vi "DAC PowerDown Step.vi"(5 "start label":string, 6 "DAC channel":u32, 7 "waveform name":string, 8 "error in":errorcluster, 11 "Digital sesssion":refnum<k15>) -> (0 "error out":errorcluster, 3 "Digital session out":refnum<k15>)   [LabVIEW 2021]
uses:
  <instrlib>/niDigital/niDigital.llb/niDigital Write Source Waveform (Broadcast U32).vi
  <instrlib>/niDigital/niDigital.llb/niDigital Burst Pattern (Pass Fail).vi
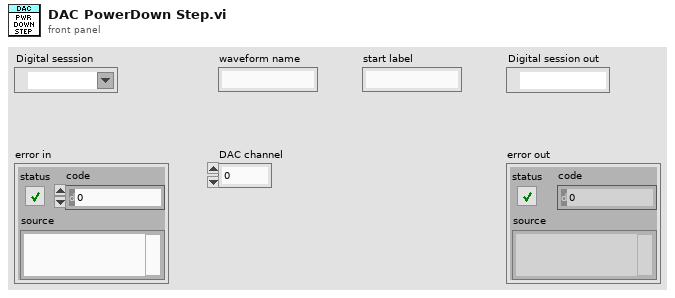
[diagram p1: front panel]
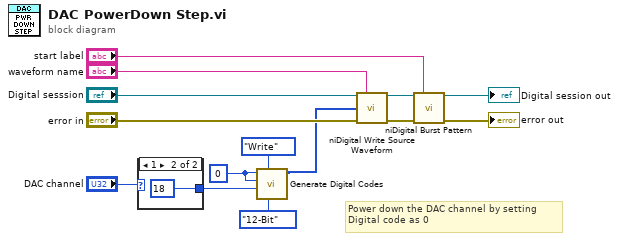
[diagram p0: block diagram]
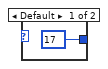
[diagram p2: hidden frame]
diagram:
  w3 = 0
  # "Power down the DAC channel by setting\nDigital code as 0"
  n1 = case shown="1" "DAC channel" {
    tunnel: [u8 17 u8 18] -> w1
    frame Default {
    }
    frame 1 {
    }
  }
  n2 = call "Generate Digital Codes.vi"("Input Code Bit"=enum16{"16-Bit", "12-Bit"}."12-Bit", "Command"=enum16{"Read", "Write"}."Write", "Address"=w1, "End code"=w3, "Start code"=w3) -> ("Digital commands"=w6:i16[])  [unwired: 4 in, 2 out]
  n3 = call-poly <instrlib>:"niDigital Write Source Waveform.vi"("instrument handle"="Digital sesssion", "waveform name"="waveform name", "waveform data"=w6, "error in"="error in") -> ("instrument handle out"=w7:refnum<k15>, "error out"=w8:errorcluster)  [unwired: 10 in]
  n4 = call-poly <instrlib>:"niDigital Burst Pattern.vi"("instrument handle"=w7, "start label"="start label", "error in"=w8) -> ("instrument handle out"=→"Digital session out":refnum<k15>, "error out"=→"error out":errorcluster)  [unwired: 10 in, 1 out]
